vi "LevyLab Instrument.getAll.vi"(8 "error in (no error)":errorcluster, 11 "ExampleInstrument in":refnum<class "LevyLab Instrument.lvclass">) -> (0 "error out":errorcluster, 2 "getAll":T1, 3 "ExampleInstrument out":refnum<class "LevyLab Instrument.lvclass">)   [LabVIEW 2016, in "LevyLab Instrument.lvclass"]
uses:
  LevyLab Instrument.lvclass
  C:/user/patrick/hg/levylab_inst/lvsrc/SMOs/Instrument/Instrument.lvclass
  Typedefs/LevyLab Instrument.getAll--Cluster.ctl
  SMOs/Instrument/Instrument.lvclass
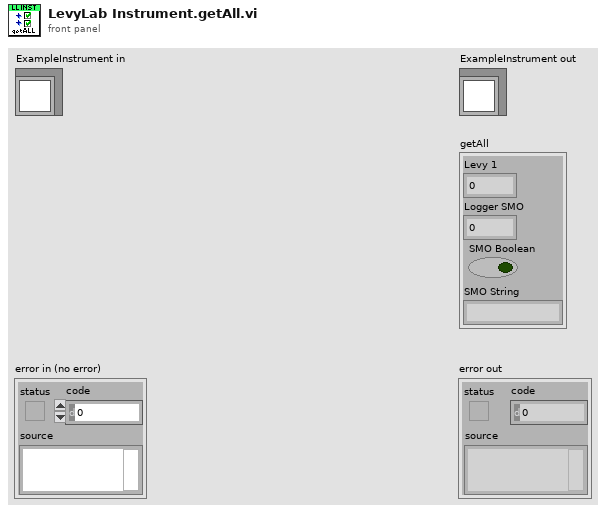
[diagram p1: front panel]
types:
  T1 = typedef "LevyLab Instrument.lvclass/LevyLab Instrument.getAll--Cluster.ctl" = cluster{"Levy 1":dbl, "Logger SMO":dbl, "SMO Boolean":bool, "SMO String":string}
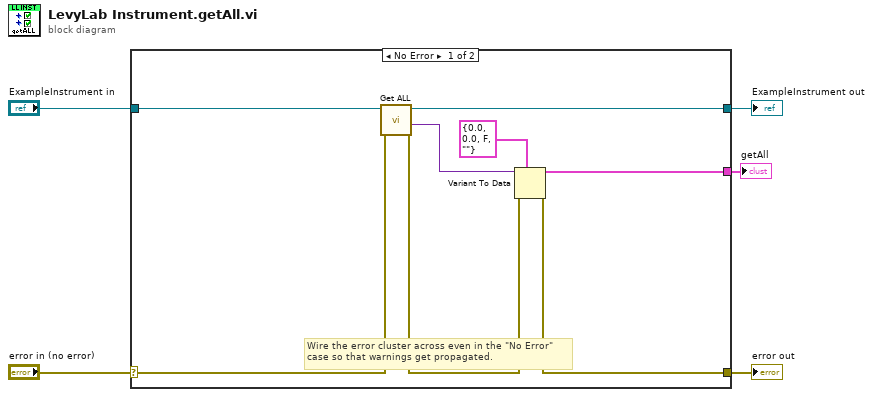
[diagram p0: block diagram]
diagram:
  n1 = case shown="No Error" "error in (no error)" {
    selector: "error in (no error)" -> [w9 w15]
    tunnel: [w7 w15] -> w4
    tunnel: [w10 w14] -> w2
    tunnel: "ExampleInstrument in" -> [w11 w14]
    tunnel: [w6 _] -> w1
    frame No Error {
      # "Wire the error cluster across even in the \"No Error\"\ncase so that warnings get propagated."
      n2 = call "Get ALL.vi"("error in (no error)"=w9, "Instrument in"=w11) -> ("error out"=w8:errorcluster, "Data out"=w13:variant, "Instrument out"=w10:refnum<class "LevyLab Instrument.lvclass">)  [unwired: 7 in]
      n3 = Variant To Data(error in=w8, type=T1 {"Levy 1"=0.0, "Logger SMO"=0.0, "SMO Boolean"=FALSE, "SMO String"=""} ("getAll"), Variant=w13) -> (data=w6:T1, error out=w7:errorcluster)
    }
    frame Error {
    }
  }
  "error out" <- w4
  "ExampleInstrument out" <- w2
  "getAll" <- w1
